vi "GraphDisplay.vi"(3 "notifier out":refnum<notifier>) -> ()   [LabVIEW 2024]
uses:
  support/Control/Array Data Constant.ctl
  Global 1.vi
panel:
  out "Data Chart":dbl[][](graph)
  in  "Listbox":i32[](listbox)
  in  "Close":bool
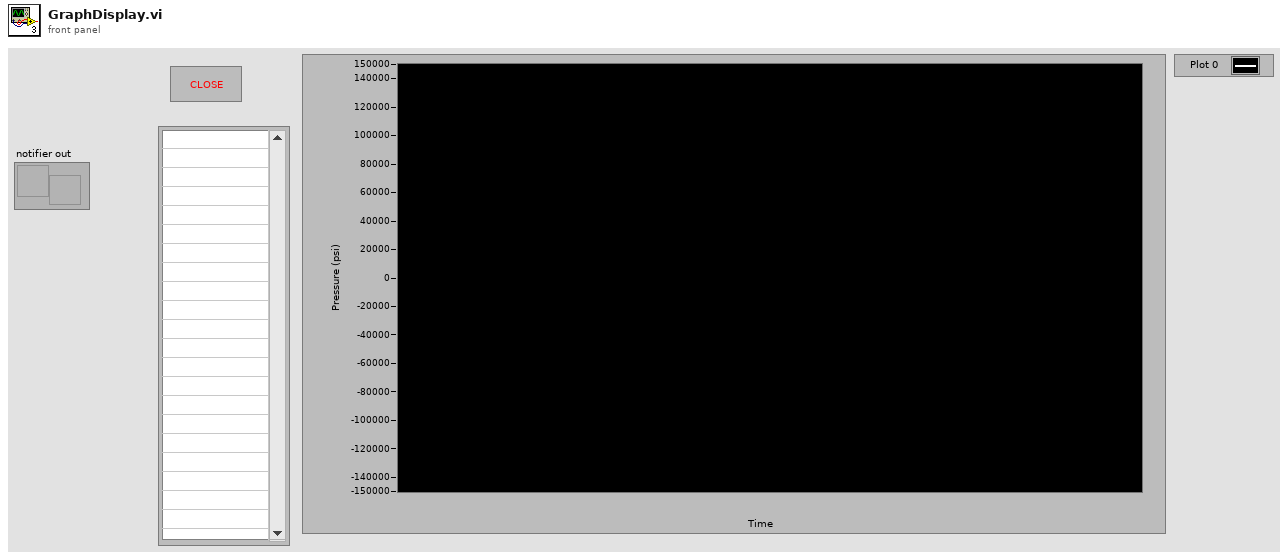
[diagram p1: front panel]
types:
  T1 = typedef "Calibration Configuration.ctl" = cluster{"ai Calibration Slope":dbl[], "ai Calibration Offset":dbl[], "ai Sensor Names ":string[], "tc Sensor Names":string[], "di Sensor Names":string[], "do Sensor Names":string[], "bc Sensor Names":string[], "ai Sensor Units":string[], "tc Sensor Units":string[], "bc Sensor Units":string[]}
  T2 = typedef "Array Data Constant.ctl" = cluster{"AI":dbl[], "TC":dbl[], "BC":dbl[], "DI":dbl[], "t (UTC)":dbl}
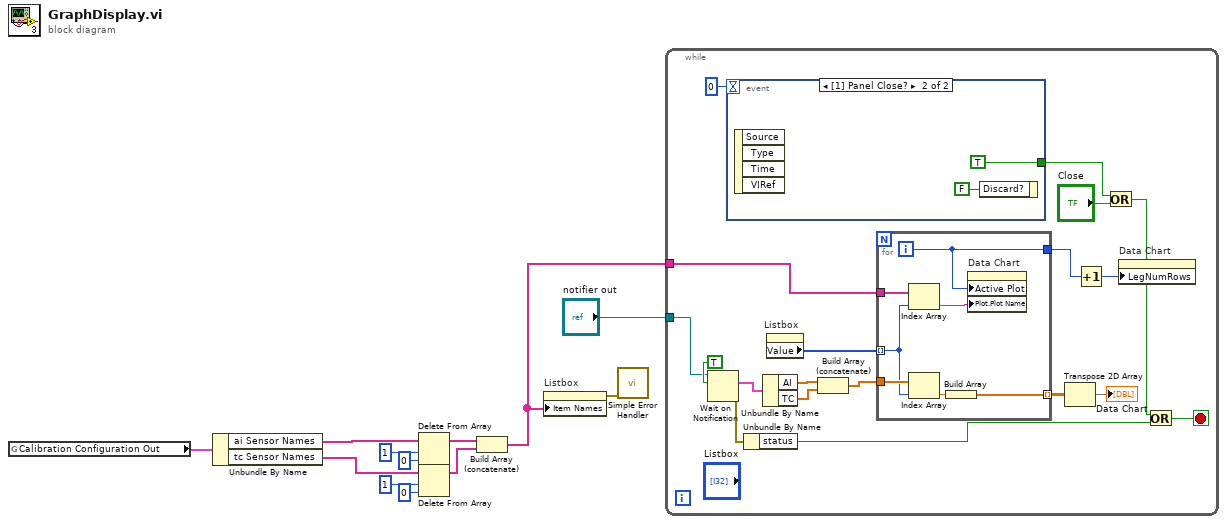
[diagram p0: block diagram]
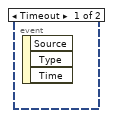
[diagram p2: hidden frame]
diagram:
  n1 = global read "Global 1.vi" "Calibration Configuration Out"() -> (w11:T1)
  n2 = Unbundle By Name(w11) -> ("ai Sensor Names"=w8:string[], "tc Sensor Names"=w3:string[])
  n3 = Delete From Array(array=w8, length=1, index=0) -> (array with subset deleted=w7:string[])  [unwired: 1 out]
  n4 = Delete From Array(array=w3, length=1, index=0) -> (array with subset deleted=w1:string[])  [unwired: 1 out]
  n5 = Build Array (concatenate)(w7, w1) -> (w2:string[])
  n6 = property on="Listbox" class="LstBox (strict)"("Item Names"=w2) -> (error out=w6:errorcluster)  [unwired: 2 in, 1 out]
  n7 = call <vilib>:"Simple Error Handler.vi"("error in (no error)"=w6) -> ()  [unwired: 4 in, 5 out]
  n8 = while {
    tunnel: "notifier out" -> [w26]
    tunnel: w2 -> [w18]
    stop <- w24 stop-if-true
    n9 = Wait on Notification(notifier=w26, ignore previous (F)=TRUE) -> (notification=w22:T2, error out=w28:errorcluster)  [unwired: 2 in, 2 out]
    n10 = event shown="[1] Panel Close?" {
      selector: _ -> [_ _]
      dyn-events: _ -> [_ _]
      timeout: 0 -> [_ _]
      tunnel: [_ TRUE] -> w30
      event Timeout {
        n11 = event-data() -> ()  [unwired: 1 in, 3 out]
      }
      event Panel Close? {
        n12 = event-data() -> ()  [unwired: 1 in, 4 out]
        n13 = event-data("Discard?"=FALSE) -> ()  [unwired: 1 in, 1 out]
      }
    }
    n14 = Unbundle By Name(w28) -> ("status"=w23:bool)
    n15 = Unbundle By Name(w22) -> ("AI"=w21:dbl[], "TC"=w14:dbl[])
    n16 = property on="Listbox" class="LstBox (strict)"() -> ("Value"=w13:i32[])  [unwired: 2 in, 2 out]
    n17 = Build Array (concatenate)(w21, w14) -> (w15:dbl[])
    n18 = for {
      tunnel: w13 -> [w35] mode=indexing
      tunnel: w15 -> [w38]
      tunnel: [w36] -> w20 mode=indexing
      tunnel: w18 -> [w34]
      tunnel: [w32] -> w17
      i -> [w32]
      n19 = Index Array(array=w34, index=w35) -> (element=w33:string)
      n20 = Index Array(array=w38, index=w35) -> (element=w37:dbl)
      n21 = Build Array(w37) -> (w36:dbl[])
      n22 = property on="Data Chart" class="WFChart (strict)"("Active Plot"=w32, "Plot.Plot Name"=w33) -> ()  [unwired: 2 in, 2 out]
    }
    n23 = Transpose 2D Array(2D array=w20) -> (transposed array=→"Data Chart":dbl[][])
    n24 = Increment(x=w17) -> (x+1=w16:i32)
    n25 = Or(x=w30, y="Close") -> (x .or. y?=w25:bool)
    n26 = property on="Data Chart" class="WFChart (strict)"("LegNumRows"=w16) -> ()  [unwired: 2 in, 2 out]
    n27 = Or(x=w25, y=w23) -> (x .or. y?=w24:bool)
  }
